vi "Control Read 2.vi"(4 "error in (no error)":errorcluster, 6 "Container State":T2, 7 "Display State In":T1) -> (0 "error out":errorcluster, 2 "Value":refnum<k24>, 3 "Display State Out":T1)   [LabVIEW 2020, in "WebView2 XControl.lvlib" / "WebView2 Control.xctl"]
uses:
  WebView2 Control.xctl
  <vilib>/_xctls/Container State.ctl
  State.ctl
  Webview2 Lib/WebView2 Control Object/WebView2 Control.lvclass
  C:/Users/Simon/Documents/GitHub/LV-WebView2/Source/Libs/Microsoft.Web.WebView2.WinForms.dll
  Libs/Microsoft.Web.WebView2.WinForms.dll
  Webview2 Lib/WebView2 Control Object/Read Control.vi
  <vilib>/_xctls/XControlSupport.lvlib
panel:
  # "Replace the Value Indicator below with an Indicator of desired type.\nDo not remove this Indicator or the others from the connector pane. \nDo not change the connector pane pattern.\nThe Value Indicator should always be the second terminal from top on the output side in the connector pane."
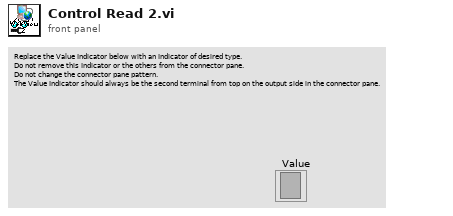
[diagram p1: front panel]
types:
  T1 = typedef "WebView2 XControl.lvlib/WebView2 Control.xctl/State.ctl" = cluster{"Control Object Ref":refnum<data-value>}
  T2 = typedef "XControlSupport.lvlib/Container State.ctl" = cluster{"Indicator?":bool, "Run Mode?":bool, " Refnum":refnum<vi>}
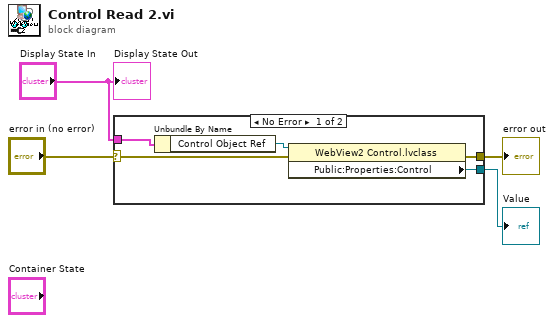
[diagram p0: block diagram]
diagram:
  n1 = case shown="No Error" "error in (no error)" {
    selector: "error in (no error)" -> [w9 w10]
    tunnel: [w5 _] -> w4
    tunnel: [w7 w10] -> w2
    tunnel: "Display State In" -> [w8 _]
    frame No Error {
      n2 = Unbundle By Name(w8) -> ("Control Object Ref"=w6:refnum<data-value>)
      n3 = property class="WebView2 Control.lvclass"(reference=w6, error in=w9) -> (error out=w7:errorcluster, "Public:Properties:Control"=w5:refnum<k24>)  [unwired: 1 out]
    }
    frame Error {
    }
  }
  "error out" <- w2
  "Value" <- w4
  "Display State Out" <- "Display State In"
